vi "Is Identity Matrix.vi"() -> ()   [LabVIEW 2019]
uses:
  <vilib>/silver_ctls/ArrayMatrixCluster/Real Matrix NI_Silver.ctl
panel:
  in  "Real Matrix":T1
  out "dan wei zhen?":bool
  out "String":string
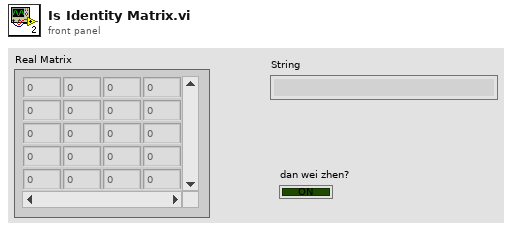
[diagram p1: front panel]
types:
  T1 = typedef "Real Matrix NI_Silver.ctl" = dbl[][]
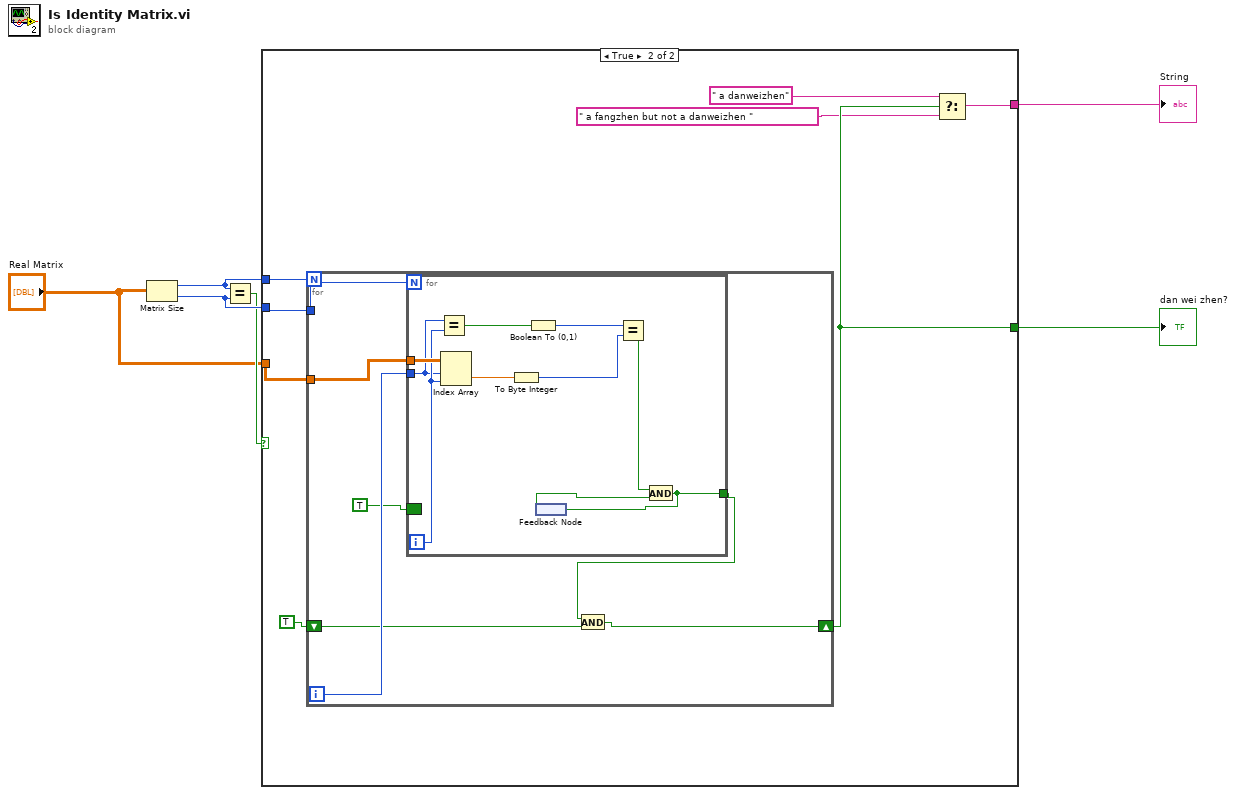
[diagram p0: block diagram]
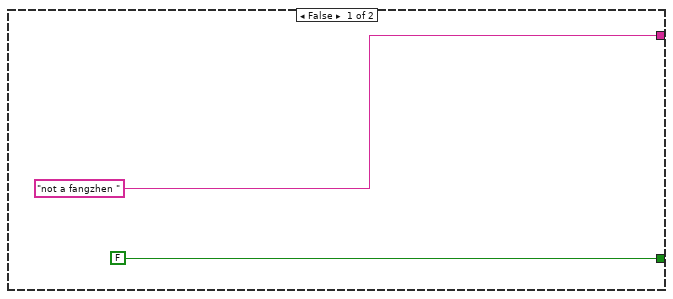
[diagram p2: hidden frame]
diagram:
  n1 = Matrix Size(0:"Real Matrix") -> (1:w5:i32, 2:w4:i32)
  n2 = Equal?(x=w5, y=w4) -> (x = y?=w2:bool)
  n3 = case shown="True" w2 {
    tunnel: ["not a fangzhen " w12] -> w6
    tunnel: w5 -> [_ w16]
    tunnel: w4 -> [_ w15]
    tunnel: [FALSE w11] -> w3
    tunnel: "Real Matrix" -> [_ w14]
    frame False {
    }
    frame True {
      n4 = for {
        N: w16 -> [_]
        tunnel: w15 -> [w23]
        tunnel: w14 -> [w22]
        shift-right: [w19] -> w11
        shift-left: TRUE -> [w20]
        i -> [w21]
        n5 = for {
          N: w23 -> [_]
          tunnel: w22 -> [w33]
          tunnel: w21 -> [w27]
          border: TRUE -> [_]
          tunnel: [w26] -> w18
          i -> [w28]
          n6 = Equal?(x=w27, y=w28) -> (x = y?=w32:bool)
          n7 = Index Array(array=w33, index (row)=w27, index (col)=w28) -> (element=w30:dbl)
          n8 = To Byte Integer(number=w30) -> (8bit integer=w29:i8)
          n9 = Boolean To (0,1)(Boolean=w32) -> (0, 1=w31:i16)
          n10 = feedback #1() -> (w24:bool)
          n11 = Equal?(x=w31, y=w29) -> (x = y?=w25:bool)
          n12 = And(x=w25, y=w24) -> (x .and. y?=w26:bool)
          n13 = feedback-in #1(w26) -> ()
        }
        n14 = And(x=w18, y=w20) -> (x .and. y?=w19:bool)
      }
      n15 = Select(t=" a danweizhen", s=w11, f=" a fangzhen but not a danweizhen ") -> (s? t:f=w12:string)
    }
  }
  "String" <- w6
  "dan wei zhen?" <- w3
